vi "Check If Duplicate Name.vi"(9 "Type Name Library File Path":map{string, map{string, path}}(c390), 10 "Template Library File Path":path) -> (2 "Duplicate?":bool)   [LabVIEW 2021, in "_Template.lvlib" / "_Template.lvclass"]
uses:
  _Template.lvclass
  _Template.lvclass/_Template.ctl
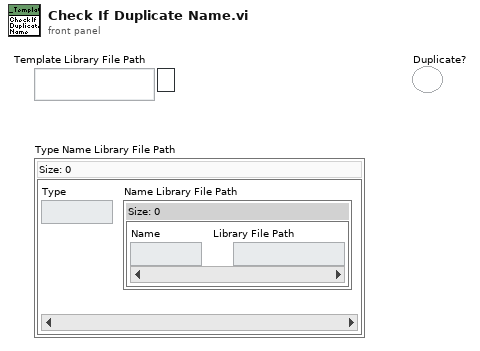
[diagram p1: front panel]
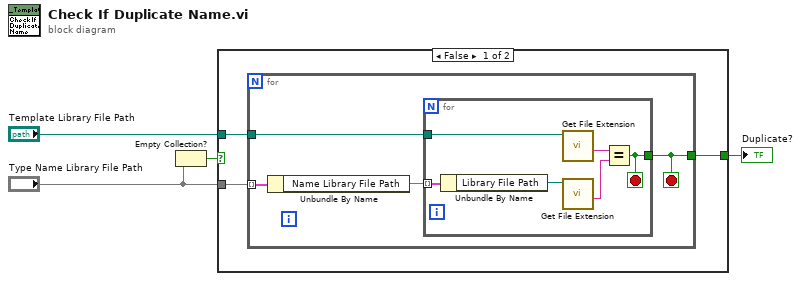
[diagram p0: block diagram]
diagram:
  n1 = Empty Collection?(1:"Type Name Library File Path") -> (0:w4:bool)
  n2 = case shown="False" w4 {
    tunnel: "Template Library File Path" -> [w7 _]
    tunnel: [w5 _] -> w1
    tunnel: "Type Name Library File Path" -> [w6 _]
    frame False {
      n3 = for {
        tunnel: w6 -> [w11] mode=indexing
        tunnel: w7 -> [w9]
        tunnel: [w8] -> w5
        stop <- w8 stop-if-true
        n4 = Unbundle By Name(w11) -> ("Name Library File Path"=w10:map{string, path})
        n5 = for {
          tunnel: w10 -> [w17] mode=indexing
          tunnel: w9 -> [w15]
          tunnel: [w16] -> w8
          stop <- w16 stop-if-true
          n6 = Unbundle By Name(w17) -> ("Library File Path"=w13:path)
          n7 = call <vilib>:"Get File Extension.vi"("file"=w15) -> ("filename without extension"=w14:string)  [unwired: 6 in, 4 out]
          n8 = call <vilib>:"Get File Extension.vi"("file"=w13) -> ("filename without extension"=w12:string)  [unwired: 6 in, 4 out]
          n9 = Equal?(x=w14, y=w12) -> (x = y?=w16:bool)
        }
      }
    }
    frame True {
    }
  }
  "Duplicate?" <- w1
